vi "Set Print.vi"(8 "error in (no error)":errorcluster, 10 "On?":bool=TRUE, 11 "Main.lvlib:Main.lvclass":refnum<class "Main.lvclass">) -> (0 "error out":errorcluster, 3 "Actor out":refnum<class "Actor.lvclass">)   [LabVIEW 2018]
uses:
  MFC Actor/MFC Messages/Set Print Msg/Set Print Msg.lvclass
  Feeder Actor/Feeder Messages/Set Feeder Msg/Set Feeder Msg.lvclass
  <vilib>/ActorFramework/Message Enqueuer/Message Enqueuer.lvclass
  Main.lvclass
  C:/Program Files/National Instruments/LabVIEW 2018/vi.lib/MGI/Panel Manager/Panel Actor/Panel Actor/Panel Actor.lvclass
  C:/Program Files/National Instruments/LabVIEW 2018/vi.lib/MGI/Monitored Actor/Monitored Actor/Monitored Actor/Monitored Actor.lvclass
  C:/Program Files/National Instruments/LabVIEW 2018/vi.lib/ActorFramework/Actor/Actor.lvclass
  <vilib>/ActorFramework/Actor/Actor.lvclass
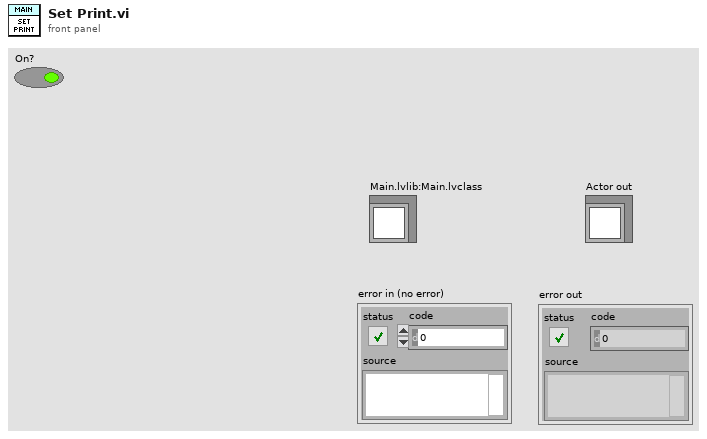
[diagram p1: front panel]
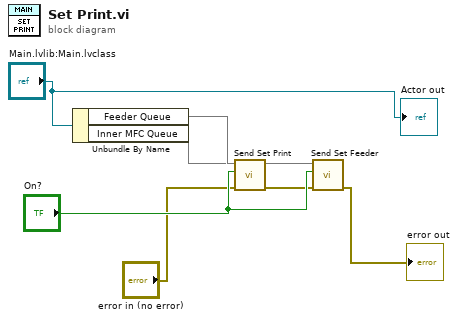
[diagram p0: block diagram]
diagram:
  n1 = Unbundle By Name("Main.lvlib:Main.lvclass") -> ("Feeder Queue"=w7, "Inner MFC Queue"=w6)
  n2 = call "Send Set Print.vi"("error in (no error)"="error in (no error)", "On?"="On?", "Message Enqueuer in"=w6) -> ("error out"=w3:errorcluster)  [unwired: 7 in, 1 out]
  n3 = call "Send Set Feeder.vi"("error in (no error)"=w3, "State"="On?", "Message Enqueuer in"=w7) -> ("error out"=→"error out":errorcluster)  [unwired: 7 in, 1 out]
  "Actor out" <- "Main.lvlib:Main.lvclass"
